vi "BurstTrain-Init (Continuous).vi"(0 "Ramp (ms)":dbl, 5 "Duration (ms)":dbl, 7 "Start Rate (Hz)":dbl, 9 "Fs (Hz)":dbl, 11 "error in (no error)":errorcluster) -> (4 "Initial State":T1, 15 "error out":errorcluster)   [LabVIEW 2015]
uses:
  Burst Train-Continuous State.ctl
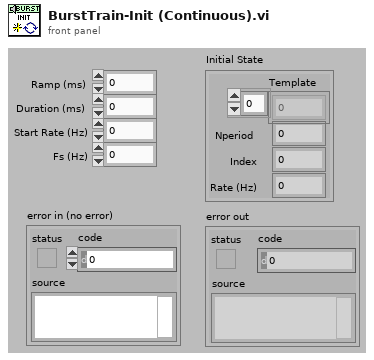
[diagram p1: front panel]
types:
  T1 = typedef "Burst Train-Continuous State.ctl" = cluster{"Template":dbl[], "Nperiod":i32, "Index":i32, "Rate (Hz)":dbl}
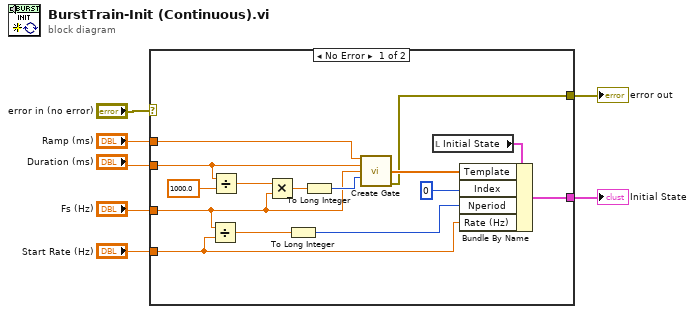
[diagram p0: block diagram]
diagram:
  n1 = case shown="No Error" "error in (no error)" {
    selector: "error in (no error)" -> [_ w23]
    tunnel: [w16 w23] -> w6
    tunnel: "Fs (Hz)" -> [w8 _]
    tunnel: [w21 _] -> w4
    tunnel: "Start Rate (Hz)" -> [w14 _]
    tunnel: "Ramp (ms)" -> [w15 _]
    tunnel: "Duration (ms)" -> [w13 _]
    frame No Error {
      n2 = Divide(x=w8, y=w14) -> (x/y=w19:dbl)
      n3 = Divide(x=w13, y=1000.0) -> (x/y=w11:dbl)
      n4 = Multiply(x=w11, y=w8) -> (x*y=w10:dbl)
      n5 = To Long Integer(number=w19) -> (32bit integer=w18:i32)
      n6 = To Long Integer(number=w10) -> (32bit integer=w9:i32)
      n7 = call "Create Gate.vi"("Ramp (ms)"=w15, "Duration (ms)"=w13, "Sampling Rate (Hz)"=w8, "Npts"=w9) -> ("Gate"=w17:dbl[], "error out"=w16:errorcluster)  [unwired: 10 in]
      n8 = local read "Initial State"() -> (w22:T1)
      n9 = Bundle By Name(cluster=w22, "Template"=w17, "Index"=0, "Nperiod"=w18, "Rate (Hz)"=w14) -> (w21:T1)
    }
    frame Error {
    }
  }
  "error out" <- w6
  "Initial State" <- w4
